vi "33XXX源设置.vi"(6 "步长":i32, 8 "error in":errorcluster, 10 "设置":string[](array[string])=["160", "10", "0.02", "0.02", "0.1", "10", "J5", "J6"], 11 "VISA引用句柄输入":refnum<visa-resource-name>) -> (0 "error out":errorcluster, 3 "VISA resource name out":refnum<visa-resource-name>)   [LabVIEW 2015]
uses:
  Agilent 3352X Series/Agilent 3352X Series.lvlib
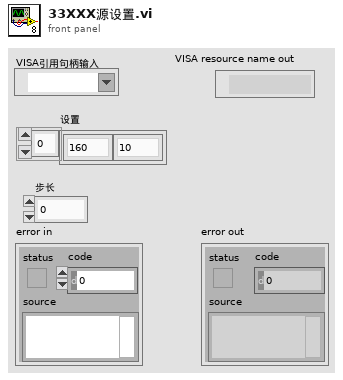
[diagram p1: front panel]
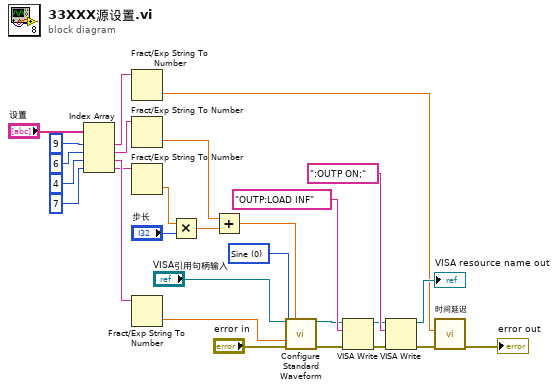
[diagram p0: block diagram]
diagram:
  w1 = 0 items=["Sine"=0, "Square"=1, "Ramp"=2, "Noise"=3, "DC"=4, "Triangle"=5, "Pulse"=6, "Sinc"=11, "D-Lorentz"=12, "Gaussian"=13, "Expo Fall"=14, "Expo Rise"=15, "Haversine"=16] ("Waveform Function (0: Sine)")
  n1 = Index Array(array="设置", index #1=9 ("索引"), index #2=6 ("索引 (行)"), index #3=4 ("索引"), index #4=7 ("索引")) -> (element #1=w12:string, element #2=w27:string, element #3=w24:string, element #4=w22:string)
  n2 = Fract/Exp String To Number(string=w12) -> (number=w11:dbl)  [unwired: 3 in, 1 out]
  n3 = Fract/Exp String To Number(string=w27) -> (number=w20:dbl)  [unwired: 3 in, 1 out]
  n4 = Fract/Exp String To Number(string=w22) -> (number=w21:dbl)  [unwired: 3 in, 1 out]
  n5 = Fract/Exp String To Number(string=w24) -> (number=w9:dbl)  [unwired: 3 in, 1 out]
  n6 = Multiply(x=w21, y="步长") -> (x*y=w19:dbl)
  n7 = Add(x=w20, y=w19) -> (x+y=w10:dbl)
  n8 = call "Configure Standard Waveform.vi"("VISA resource name"="VISA引用句柄输入", "Amplitude (0.1 Vpp)"=w10, "Waveform Function (0: Sine)"=w1, "Frequency/Sample Rate/Bandwidth (1000 Hz)"=w9, "error in (no error)"="error in") -> ("VISA resource name out"=w5:refnum<visa-resource-name>, "error out"=w4:errorcluster)  [unwired: 9 in]
  n9 = VISA Write(VISA resource name=w5, write buffer="OUTP:LOAD INF", error in (no error)=w4) -> (VISA resource name out=w3:refnum<visa-resource-name>, error out=w2:errorcluster)  [unwired: 1 out]
  n10 = VISA Write(VISA resource name=w3, write buffer=":OUTP ON;" ("true string"), error in (no error)=w2) -> (VISA resource name out=→"VISA resource name out":refnum<visa-resource-name>, error out=w15:errorcluster)  [unwired: 1 out]
  n11 = call "时间延迟"("error in (no error)"=w15, "Delay Time (s)"=w11) -> ("error out"=→"error out":errorcluster)  [unwired: 9 in]
